vi "Write driveMode.vi"(8 "error in (no error)":errorcluster, 10 "driveMode":enum16{"velocityMode", "torqueMode", ""}(ring), 11 "MotorController in":refnum<class "MotorController.lvclass">) -> (0 "error out":errorcluster, 3 "MotorController out":refnum<class "MotorController.lvclass">)   [LabVIEW 2017, in "MotorController.lvclass"]
uses:
  MotorController.lvclass
  MotorController.lvclass/MotorController.ctl
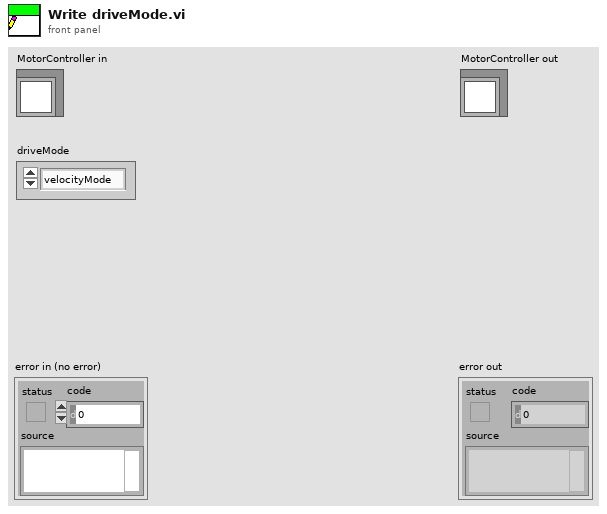
[diagram p1: front panel]
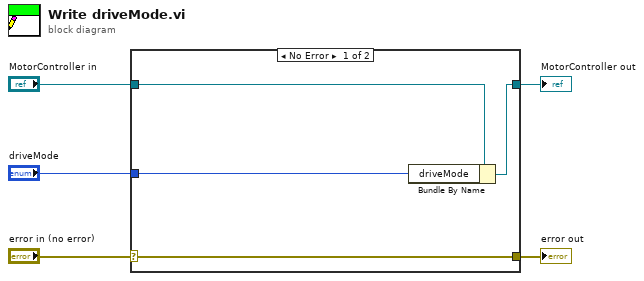
[diagram p0: block diagram]
diagram:
  n1 = case shown="No Error" "error in (no error)" {
    selector: "error in (no error)" -> [w9 w10]
    tunnel: [w9 w10] -> w4
    tunnel: [w7 w11] -> w2
    tunnel: "MotorController in" -> [w8 w11]
    tunnel: "driveMode" -> [w6 _]
    frame No Error {
      n2 = Bundle By Name(cluster=w8, "driveMode"=w6) -> (w7:refnum<class "MotorController.lvclass">)
    }
    frame Error {
    }
  }
  "error out" <- w4
  "MotorController out" <- w2
